vi "ReadNmeaData.vi"(8 "error in":errorcluster, 9 "Airmar Wind Queue Cluster":T1, 10 "GPS-Compass Queue Cluster":T2, 11 "Serial Port":refnum<visa-resource-name>) -> (0 "error out":errorcluster)   [LabVIEW 2013]
uses:
  Data/TypeDefs/GPS-Compass Queue Cluster.ctl
  Data/TypeDefs/UTM Location.ctl
  Data/TypeDefs/WindData Queue Cluster.ctl
panel:
  out "Pitch 2":dbl
  out "Roll 2":dbl
  out "Boat Direction 2":dbl
  out "Pitch":dbl
  out "Roll":dbl
  out "Relative Wind Direction":dbl
  out "Wind Speed (m/s)":dbl
  out "Absolute Wind Direction":dbl
  out "Rate Of Turn (deg/s)":dbl
  out "Boat Direction":dbl
  out "Boat Velocity Direction":dbl
  out "Boat Speed":dbl
  out "Longitude":dbl
  out "Latitude":dbl
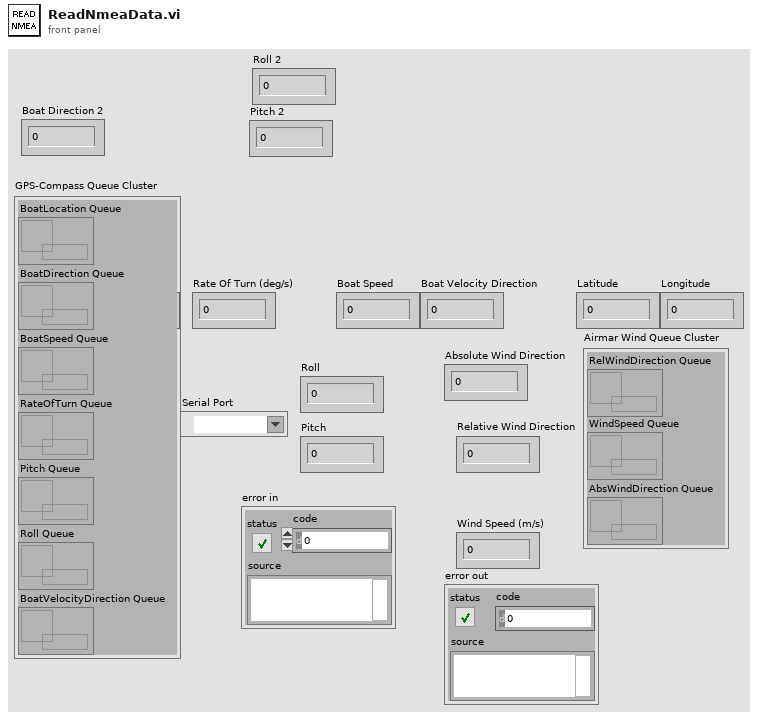
[diagram p1: front panel]
types:
  T1 = typedef "WindData Queue Cluster.ctl" = cluster{"RelWindDirection Queue":refnum<queue>, "WindSpeed Queue":refnum<queue>, "AbsWindDirection Queue":refnum<queue>}
  T2 = typedef "GPS-Compass Queue Cluster.ctl" = cluster{"BoatLocation Queue":refnum<queue>, "BoatDirection Queue":refnum<queue>, "BoatSpeed Queue":refnum<queue>, "RateOfTurn Queue":refnum<queue>, "Pitch Queue":refnum<queue>, "Roll Queue":refnum<queue>, "BoatVelocityDirection Queue ":refnum<queue>}
  T3 = typedef "UTM Location.ctl" = cluster{"UTM Zone":dbl, "Hemisphere":enum16{"North", "South"}, "East":dbl, "North":dbl}
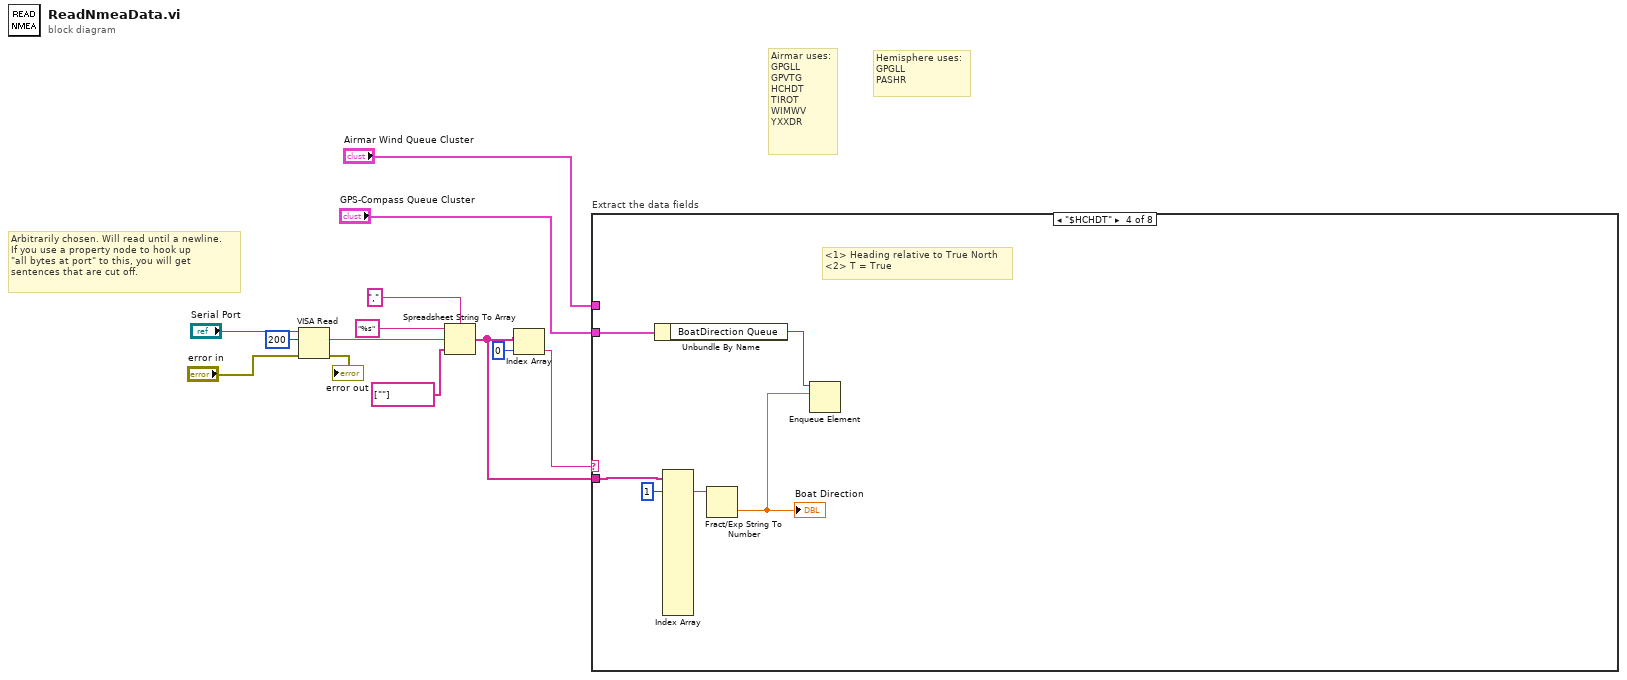
[diagram p0: block diagram]
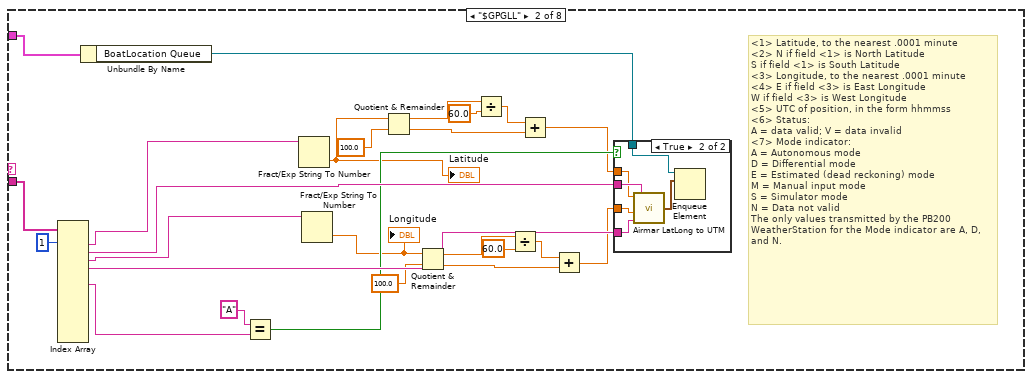
[diagram p3: hidden frame]
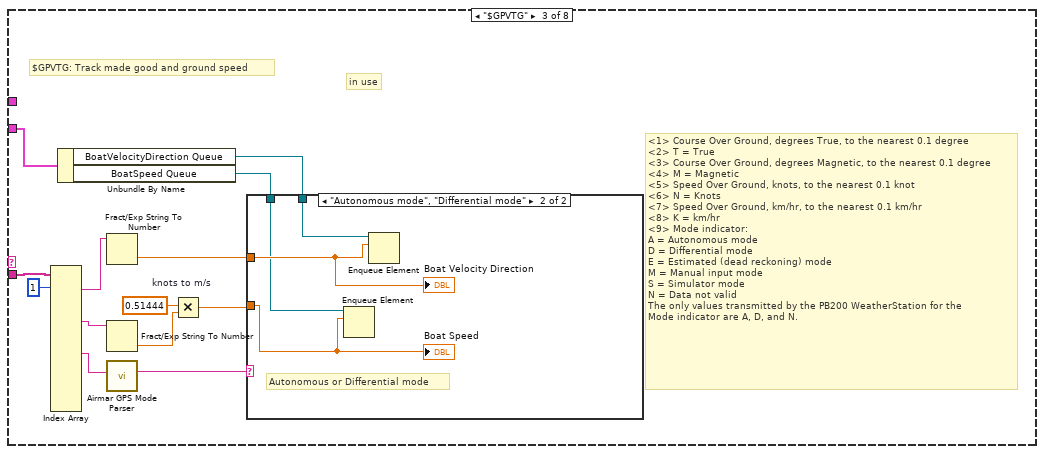
[diagram p5: hidden frame]
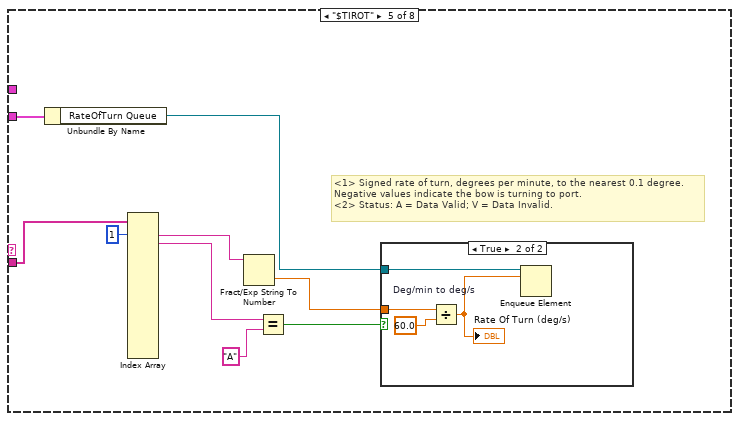
[diagram p7: hidden frame]
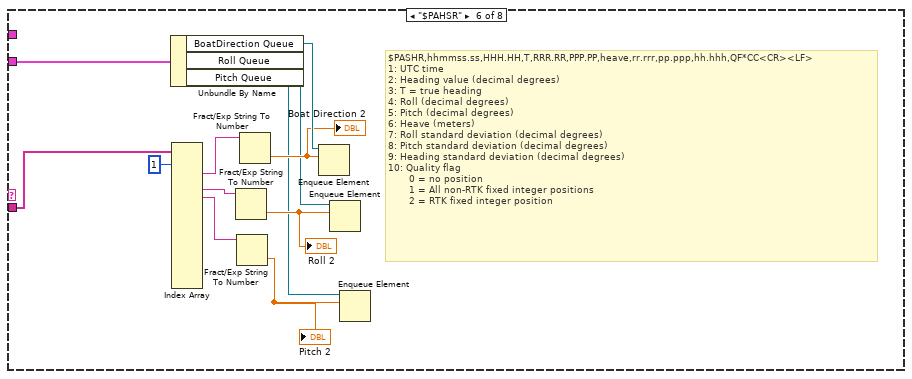
[diagram p9: hidden frame]
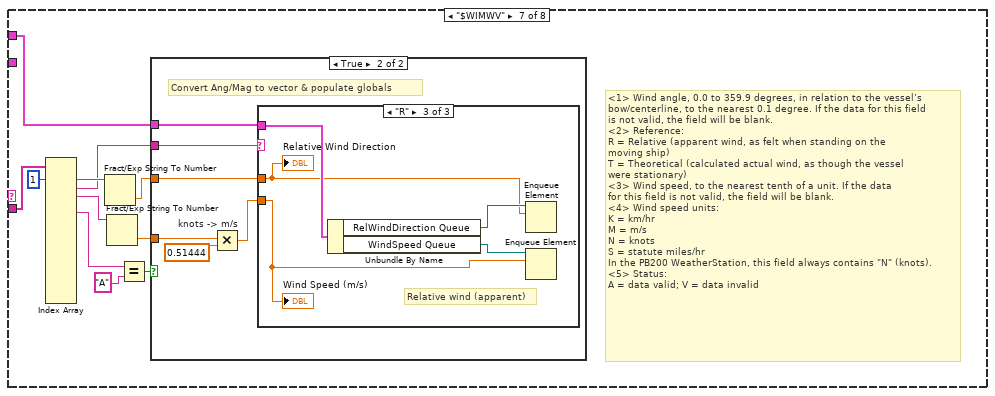
[diagram p10: hidden frame]
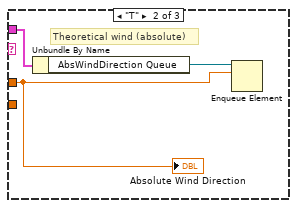
[diagram p13: hidden frame]
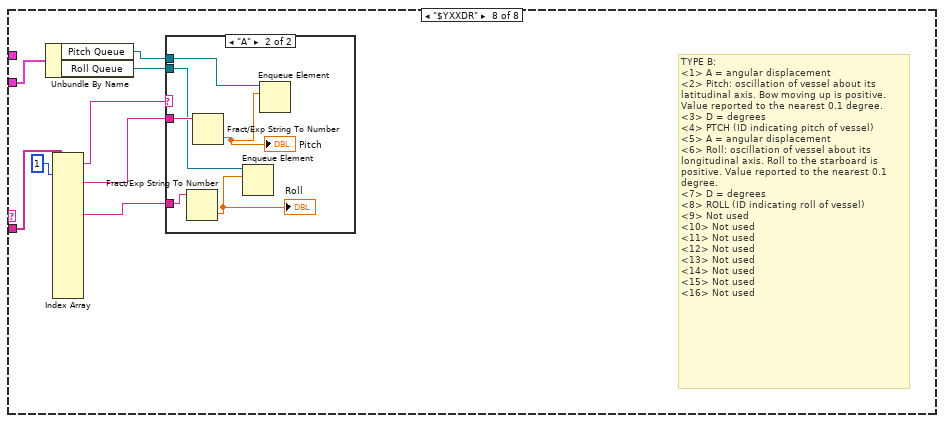
[diagram p14: hidden frame]
diagram:
  # "Hemisphere uses:\nGPGLL\nPASHR"
  # "Airmar uses:\nGPGLL\nGPVTG\nHCHDT\nTIROT\nWIMWV\nYXXDR"
  # "Arbitrarily chosen. Will read until a newline.\nIf you use a property node to hook up\n\"all bytes at port\" to this, you will get \nsentences that are cut off."
  n1 = VISA Read(VISA resource name="Serial Port", byte count=u32 200, error in (no error)="error in") -> (read buffer=w10:string, error out=→"error out":errorcluster)  [unwired: 2 out]
  n2 = Spreadsheet String To Array(delimiter (Tab)=",", format string="%s", spreadsheet string=w10, array type (2D Dbl)=string[] [""]) -> (array=w6:string[])
  n3 = Index Array(array=w6, index=0) -> (element=w4:string)
  n4 = case "Extract the data fields" shown="\"$HCHDT\"" w4 {
    tunnel: w6 -> [_ w37 w57 w67 w74 w82 w103 w125]
    tunnel: "GPS-Compass Queue Cluster" -> [_ w15 w47 w64 w69 w81 _ w120]
    tunnel: "Airmar Wind Queue Cluster" -> [_ _ _ _ _ _ w93 _]
    frame Default {
      # "Unknown sentence."
    }
    frame "$GPGLL" {
      # "<1> Latitude, to the nearest .0001 minute\n<2> N if field <1> is North Latitude\nS if field <1> is South Latitude\n<3> Longitude, to the nearest .0001 minute\n<4> E if field <3> is East Longitude\nW if field <3> is West Longitude\n<5> UTC of position, in the form hhmmss\n<6> Status:\nA = data valid; V = data invalid\n<7> Mode indicator:\nA = Autonomous mode\nD = Differential mode\nE = Estimated (dead reckoning) mode\nM = Manual input mode\nS = Simulator mode\nN = Data not valid\nThe only values transmitted by the PB200 WeatherStation for the Mode indicator are A, D, and N."
      n5 = Index Array "Index Array"(array=w37, index #1=1 ("index")) -> (element #1=w36:string, element #2=w35:string, element #3=w34:string, element #4=w33:string, element #6=w32:string)  [unwired: 12 in, 8 out]
      n6 = Unbundle By Name(w15) -> ("BoatLocation Queue"=w14:refnum<queue>)
      n7 = Equal?(x="A" ("y"), y=w32) -> (x = y?=w30:bool)
      n8 = Fract/Exp String To Number(string=w36) -> (number=w24:dbl)  [unwired: 3 in, 1 out]
      "Latitude" <- w24
      n9 = Fract/Exp String To Number(string=w34) -> (number=w17:dbl)  [unwired: 3 in, 1 out]
      "Longitude" <- w17
      n10 = Quotient & Remainder(x=w24, y=100.0) -> (x-y*floor(x/y)=w28:dbl, floor(x/y)=w25:dbl)
      n11 = Quotient & Remainder(x=w17, y=100.0) -> (x-y*floor(x/y)=w21:dbl, floor(x/y)=w19:dbl)
      n12 = Divide(x=w28, y=60.0) -> (x/y=w26:dbl)
      n13 = Divide(x=w21, y=60.0) -> (x/y=w20:dbl)
      n14 = Add(x=w26, y=w25) -> (x+y=w23:dbl)
      n15 = Add(x=w20, y=w19) -> (x+y=w18:dbl)
      n16 = case shown="True" w30 {
        tunnel: w35 -> [_ w44]
        tunnel: w18 -> [_ w43]
        tunnel: w33 -> [_ w42]
        tunnel: w23 -> [_ w41]
        tunnel: w14 -> [_ w40]
        frame False {
        }
        frame True {
          n17 = call "Airmar LatLong to UTM.vi"("East/West"=w42, "Longitude"=w43, "North/South"=w44, "Latitude"=w41) -> ("Robot UTM Location"=w39:T3)
          n18 = Enqueue Element(queue=w40, element=w39) -> ()  [unwired: 2 in, 3 out]
        }
      }
    }
    frame "$GPVTG" {
      # "<1> Course Over Ground, degrees True, to the nearest 0.1 degree\n<2> T = True\n<3> Course Over Ground, degrees Magnetic, to the nearest 0.1 degree\n<4> M = Magnetic\n<5> Speed Over Ground, knots, to the nearest 0.1 knot\n<6> N = Knots\n<7> Speed Over Ground, km/hr, to the nearest 0.1 km/hr\n<8> K = km/hr\n<9> Mode indicator:\nA = Autonomous mode\nD = Differential mode\nE = Estimated (dead reckoning) mode\nM = Manual input mode\nS = Simulator mode\nN = Data not valid\nThe only values transmitted by the PB200 WeatherStation for the\nMode indicator are A, D, and N."
      # "in use"
      # "$GPVTG: Track made good and ground speed"
      n19 = Index Array(array=w57, index #1=1 ("index")) -> (element #1=w55:string, element #5=w54:string, element #9=w53:string)  [unwired: 15 in, 13 out]
      n20 = Unbundle By Name(w47) -> ("BoatVelocityDirection Queue"=w46:refnum<queue>, "BoatSpeed Queue"=w45:refnum<queue>)
      n21 = Fract/Exp String To Number(string=w55) -> (number=w52:dbl)  [unwired: 3 in, 1 out]
      n22 = Fract/Exp String To Number(string=w54) -> (number=w50:dbl)  [unwired: 3 in, 1 out]
      n23 = call "Airmar GPS Mode Parser.vi"("GPS Mode (Char)"=w53) -> ("GPS Mode (Description)"=w48:string)  [unwired: 6 in]
      n24 = Multiply "knots to m/s"(x=0.51444 ("y"), y=w50) -> (x*y=w51:dbl)
      n25 = case shown="\"Autonomous mode\", \"Differential mode\"" w48 {
        tunnel: w52 -> [_ w60]
        tunnel: w51 -> [_ w59]
        tunnel: w46 -> [_ w61]
        tunnel: w45 -> [_ w58]
        frame "Data not valid", Default {
          # "Data not valid"
        }
        frame "Autonomous mode", "Differential mode" {
          # "Autonomous or Differential mode"
          n26 = Enqueue Element(queue=w58, element=w59) -> ()  [unwired: 2 in, 3 out]
          n27 = Enqueue Element(queue=w61, element=w60) -> ()  [unwired: 2 in, 3 out]
          "Boat Velocity Direction" <- w60
          "Boat Speed" <- w59
        }
      }
    }
    frame "$HCHDT" {
      # "<1> Heading relative to True North\n<2> T = True"
      n28 = Unbundle By Name(w64) -> ("BoatDirection Queue"=w63:refnum<queue>)
      n29 = Index Array(array=w67, index #1=1 ("index")) -> (element #1=w66:string)  [unwired: 15 in, 15 out]
      n30 = Fract/Exp String To Number(string=w66) -> (number=w62:dbl)  [unwired: 3 in, 1 out]
      "Boat Direction" <- w62
      n31 = Enqueue Element(queue=w63, element=w62) -> ()  [unwired: 2 in, 3 out]
    }
    frame "$TIROT" {
      # "<1> Signed rate of turn, degrees per minute, to the nearest 0.1 degree.\nNegative values indicate the bow is turning to port.\n<2> Status: A = Data Valid; V = Data Invalid."
      n32 = Unbundle By Name(w69) -> ("RateOfTurn Queue"=w68:refnum<queue>)
      n33 = Index Array(array=w74, index #1=1 ("index")) -> (element #1=w73:string, element #2=w71:string)  [unwired: 15 in, 14 out]
      n34 = Fract/Exp String To Number(string=w73) -> (number=w75:dbl)  [unwired: 3 in, 1 out]
      n35 = Equal?(x=w71, y="A") -> (x = y?=w76:bool)
      n36 = case shown="True" w76 {
        tunnel: w75 -> [_ w80]
        tunnel: w68 -> [_ w77]
        frame False {
        }
        frame True {
          n37 = Divide "Deg/min to deg/s"(x=w80, y=60.0) -> (x/y=w78:dbl)
          "Rate Of Turn (deg/s)" <- w78
          n38 = Enqueue Element(queue=w77, element=w78) -> ()  [unwired: 2 in, 3 out]
        }
      }
    }
    frame "$PAHSR" {
      # "$PASHR,hhmmss.ss,HHH.HH,T,RRR.RR,PPP.PP,heave,rr.rrr,pp.ppp,hh.hhh,QF*CC<CR><LF>\n1: UTC time\n2: Heading value (decimal degrees)\n3: T = true heading\n4: Roll (decimal degrees)\n5: Pitch (decimal degrees)\n6: Heave (meters)\n7: Roll standard deviation (decimal degrees)\n8: Pitch standard deviation (decimal degrees)\n9: Heading standard deviation (decimal degrees)\n10: Quality flag\n       0 = no position\n       1 = All non-RTK fixed integer positions\n       2 = RTK fixed integer position"
      n39 = Unbundle By Name(w81) -> ("BoatDirection Queue"=w91:refnum<queue>, "Roll Queue"=w87:refnum<queue>, "Pitch Queue"=w86:refnum<queue>)
      n40 = Index Array(array=w82, index #1=1 ("index")) -> (element #2=w90:string, element #4=w85:string, element #5=w84:string)  [unwired: 15 in, 13 out]
      n41 = Fract/Exp String To Number(string=w85) -> (number=w88:dbl)  [unwired: 3 in, 1 out]
      "Roll 2" <- w88
      n42 = Fract/Exp String To Number(string=w84) -> (number=w83:dbl)  [unwired: 3 in, 1 out]
      "Pitch 2" <- w83
      n43 = Fract/Exp String To Number(string=w90) -> (number=w89:dbl)  [unwired: 3 in, 1 out]
      "Boat Direction 2" <- w89
      n44 = Enqueue Element(queue=w91, element=w89) -> ()  [unwired: 2 in, 3 out]
      n45 = Enqueue Element(queue=w87, element=w88) -> ()  [unwired: 2 in, 3 out]
      n46 = Enqueue Element(queue=w86, element=w83) -> ()  [unwired: 2 in, 3 out]
    }
    frame "$WIMWV" {
      # "<1> Wind angle, 0.0 to 359.9 degrees, in relation to the vessel’s\nbow/centerline, to the nearest 0.1 degree. If the data for this field\nis not valid, the field will be blank.\n<2> Reference:\nR = Relative (apparent wind, as felt when standing on the\nmoving ship)\nT = Theoretical (calculated actual wind, as though the vessel\nwere stationary)\n<3> Wind speed, to the nearest tenth of a unit. If the data\nfor this field is not valid, the field will be blank.\n<4> Wind speed units:\nK = km/hr\nM = m/s\nN = knots\nS = statute miles/hr\nIn the PB200 WeatherStation, this field always contains \"N\" (knots).\n<5> Status:\nA = data valid; V = data invalid"
      n47 = Index Array(array=w103, index #1=1 ("index")) -> (element #1=w101:string, element #2=w98:string, element #3=w100:string, element #5=w99:string)  [unwired: 15 in, 12 out]
      n48 = Fract/Exp String To Number(string=w101) -> (number=w97:dbl)  [unwired: 3 in, 1 out]
      n49 = Fract/Exp String To Number(string=w100) -> (number=w96:dbl)  [unwired: 3 in, 1 out]
      n50 = Equal?(x=w99, y="A") -> (x = y?=w95:bool)
      n51 = case shown="True" w95 {
        tunnel: w96 -> [_ w106]
        tunnel: w97 -> [_ w109]
        tunnel: w98 -> [_ w108]
        tunnel: w93 -> [_ w104]
        frame False {
        }
        frame True {
          # "Convert Ang/Mag to vector & populate globals"
          n52 = Multiply "knots -> m/s"(x=w106, y=0.51444) -> (x*y=w107:dbl)
          n53 = case shown="\"R\"" w108 {
            tunnel: w107 -> [_ _ w113]
            tunnel: w109 -> [_ w110 w115]
            tunnel: w104 -> [_ w112 w117]
            frame "", Default {
            }
            frame "T" {
              # "Theoretical wind (absolute)"
              n54 = Unbundle By Name(w112) -> ("AbsWindDirection Queue"=w111:refnum<queue>)
              n55 = Enqueue Element(queue=w111, element=w110) -> ()  [unwired: 2 in, 3 out]
              "Absolute Wind Direction" <- w110
            }
            frame "R" {
              # "Relative wind (apparent)"
              n56 = Unbundle By Name(w117) -> ("RelWindDirection Queue"=w116:refnum<queue>, "WindSpeed Queue"=w114:refnum<queue>)
              n57 = Enqueue Element(queue=w116, element=w115) -> ()  [unwired: 2 in, 3 out]
              n58 = Enqueue Element(queue=w114, element=w113) -> ()  [unwired: 2 in, 3 out]
              "Relative Wind Direction" <- w115
              "Wind Speed (m/s)" <- w113
            }
          }
        }
      }
    }
    frame "$YXXDR" {
      # "TYPE B:\n<1> A = angular displacement\n<2> Pitch: oscillation of vessel about its latitudinal axis. Bow moving up is positive. Value reported to the nearest 0.1 degree.\n<3> D = degrees\n<4> PTCH (ID indicating pitch of vessel)\n<5> A = angular displacement\n<6> Roll: oscillation of vessel about its longitudinal axis. Roll to the starboard is positive. Value reported to the nearest 0.1 degree.\n<7> D = degrees\n<8> ROLL (ID indicating roll of vessel)\n<9> Not used\n<10> Not used\n<11> Not used\n<12> Not used\n<13> Not used\n<14> Not used\n<15> Not used\n<16> Not used"
      n59 = Unbundle By Name(w120) -> ("Pitch Queue"=w119:refnum<queue>, "Roll Queue"=w118:refnum<queue>)
      n60 = Index Array(array=w125, index #1=1 ("index")) -> (element #1=w124:string, element #2=w122:string, element #6=w121:string)  [unwired: 15 in, 13 out]
      n61 = case shown="\"A\"" w124 {
        tunnel: w122 -> [_ w131]
        tunnel: w121 -> [_ w130]
        tunnel: w119 -> [_ w129]
        tunnel: w118 -> [_ w127]
        frame "", Default {
        }
        frame "A" {
          n62 = Fract/Exp String To Number(string=w130) -> (number=w126:dbl)  [unwired: 3 in, 1 out]
          "Roll" <- w126
          n63 = Fract/Exp String To Number(string=w131) -> (number=w128:dbl)  [unwired: 3 in, 1 out]
          "Pitch" <- w128
          n64 = Enqueue Element(queue=w127, element=w126) -> ()  [unwired: 2 in, 3 out]
          n65 = Enqueue Element(queue=w129, element=w128) -> ()  [unwired: 2 in, 3 out]
        }
      }
    }
  }
